vi "tempLinSub.vi"(6 "initial states":dbl[](array[numeric])=[0.0, 0.0, 0.0, 0.0], 7 "output operating point":dbl[](array[numeric])=[0.0, 0.0, 0.0, 0.0, 0.0, 0.0], 9 "input operating point":dbl[](array[numeric])=[0.0], 10 "Linearized System":T1={"properties"={"Model name"="SubsystemModell.vi", "Input names"=["Fk"], "Output names"=["p''", "Postition", "Geschwindigkeit", "Winkel", "p'", "Beschleunigung"], "Input Delays"=[0.0], "Output Delays"=[0.0, 0.0, 0.0, 0.0, 0.0, 0.0], "Sampling Time"=0.0, "Notes"=""}, "A"=[[0.0, 1.0, 0.0, 0.0], [7206.125665656664, 7179.958035102217, 7183.010798141464, 7182.973797050876], [0.0, 0.0, 0.0, 1.0], [19.02607436476991, 18.95698491116097, 18.965045011594626, 18.9594467688912]], "B"=[[0.0], [7183.323444710824], [0.0], [19.020875981634738]], "C"=[[7206.125665656664, 7179.958035102217, 7183.010798141464, 7182.973797050876], [0.0, 0.0, 1.0, 0.0], [0.0, 0.0, 0.0, 1.0], [1.0, 0.0, 0.0, 0.0], [0.0, 1.0, 0.0, 0.0], [19.02607436476991, 18.95698491116097, 18.965045011594626, 18.9594467688912]], "D"=[[7183.323444710824], [0.0], [0.0], [0.0], [0.0], [19.020875981634738]], "StateNames"=["/Integrator 4", "/Integrator 3", "/Integrator 2", "/Integrator"], "Transport Delay"=[[0.0], [0.0], [0.0], [0.0], [0.0], [0.0]]} {"Transport Delay" format="%.2f"; "D" format="%#.2g"; "C" format="%#.2g"; "B" format="%#.2g"; "A" format="%#.2g"; "properties"."Sampling Time" format="%#.6p"; "properties"."Output Delays" format="%.4f"; "properties"."Input Delays" format="%.4f"}, 11 "input":dbl[](array[numeric])=[0.0]) -> (3 "output":dbl[](array[numeric]) format="%#_9g")   [LabVIEW 2013]
uses:
  <vilib>/addons/Control Design/_Model Construction/Model Typedefs.llb/CD State Space Model (MIMO).ctl
  <vilib>/addons/Control Design/_Model Construction/Model Typedefs.llb/CD General Elements.ctl
  <vilib>/Simulation/Implementation/Shared/SIMSCR Execution Mode.ctl
  <vilib>/Simulation/Scripting/Companion Diagram/SimConfigNode/SimParams.ctl
  <vilib>/Simulation/Scripting/Companion Diagram/SimConfigNode/_simSolvers.ctl
  <vilib>/Simulation/Param Hierarchy/Typedefs/SIMPH Param Control Actions.ctl
  <vilib>/Simulation/Implementation/Shared/NILVSim_ParamChanged.vi
  <vilib>/Simulation/Implementation/Shared/NILVSIM_BeginStep.vi
  <vilib>/Simulation/ContinuousLinear/Implementation/NILVSim State Space.llb/SIM State Space Direct (CD).vi
  <vilib>/Simulation/Implementation/Shared/NILVSim_Manager.vi
  <vilib>/Simulation/Implementation/Shared/NILVSim_FinalizeModel.vi
  <vilib>/Simulation/Implementation/Shared/SIM Unbundle Sim Info.vi
  <vilib>/Utility/error.llb/Clear Errors.vi
  <vilib>/Simulation/Implementation/Shared/NILVSim_GetModelError.vi
  <vilib>/Simulation/Implementation/Shared/SIM SimErrorHandler.vi
  <vilib>/Simulation/Implementation/Shared/SIM Bundle Sim Info.vi
  <vilib>/Simulation/Implementation/Shared/NILVSim_Initialize.vi
  <vilib>/Simulation/Utility/Implementation/NILVSim Get Time and IsAcceptedStep.vi
  <vilib>/Simulation/Implementation/Shared/SIMSH Read Queue.vi
  <vilib>/Simulation/Scripting/Companion Diagram/SimConfigNode/SimDog.xnode
  <vilib>/Simulation/Implementation/XNodeFramework/SimXNode/SimX.xnode
  <vilib>/addons/Control Design/_Model Construction/NI_LinSys_Model Typedefs.lvlib
  <vilib>/Simulation/Implementation/Shared/NI_SIM_Implementation.lvlib
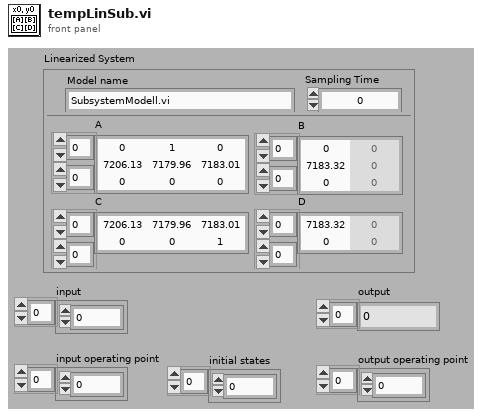
[diagram p1: front panel]
types:
  T1 = typedef "NI_LinSys_Model Typedefs.lvlib/CD State Space Model (MIMO).ctl" = cluster{"properties":T2, "A":dbl[][], "B":dbl[][], "C":dbl[][], "D":dbl[][], "StateNames":string[], "Transport Delay":dbl[][]}
  T2 = typedef "NI_LinSys_Model Typedefs.lvlib/CD General Elements.ctl" = cluster{"Model name":string, "Input names":string[], "Output names":string[], "Input Delays":dbl[], "Output Delays":dbl[], "Sampling Time":dbl, "Notes":string}
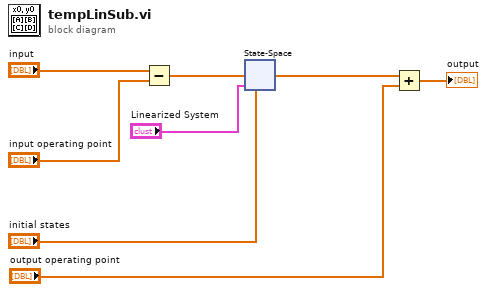
[diagram p0: block diagram]
diagram:
  n1 = Subtract(x="input", y="input operating point") -> (x-y=w3:dbl[])
  n2 = xnode ("State-Space")("input u(t)"=w3, "State-Space"="Linearized System", "initial state (x0)"="initial states") -> ("output y(t)"=w2:dbl[])  [unwired: 4 in, 1 out]
  n3 = Add(x=w2, y="output operating point") -> (x+y=→"output":dbl[])
